vi "tearDown.vi"(8 "error in (no error)":errorcluster, 11 "FrameworkSubTestSuite in":refnum<class "FrameworkSubTestSuite.lvclass">) -> (0 "error out":errorcluster, 3 "FrameworkSubTestSuite out":refnum<class "FrameworkSubTestSuite.lvclass">)   [LabVIEW 2011, in "FrameworkSubTestSuite.lvclass"]
uses:
  FrameworkSubTestSuite.lvclass
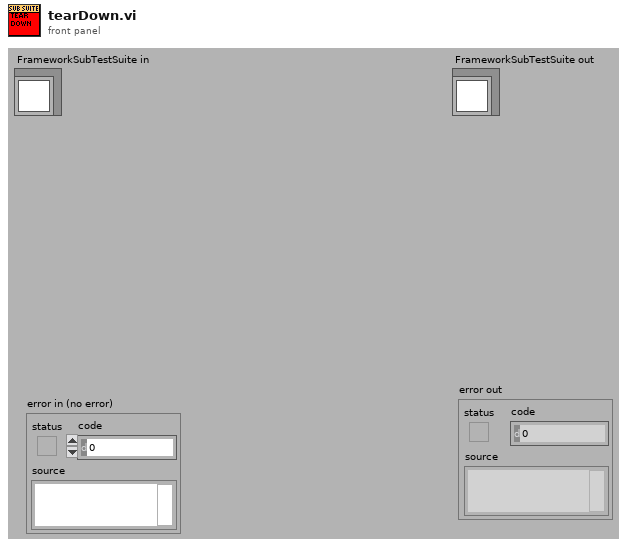
[diagram p1: front panel]
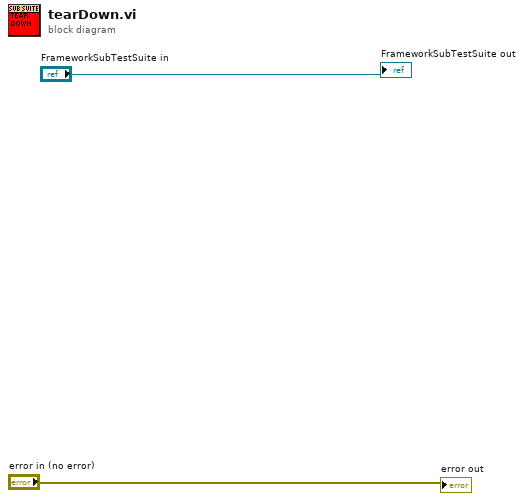
[diagram p0: block diagram]
diagram:
  "FrameworkSubTestSuite out" <- "FrameworkSubTestSuite in"
  "error out" <- "error in (no error)"
